vi "Compute Waveform.vi"(6 "signal type":T1, 8 "amplitude":dbl, 9 "phase increment":dbl, 10 "phase in":dbl, 11 "wfm size":i32) -> (2 "phase out":dbl, 3 "wfm array":dbl[](array[numeric]))   [LabVIEW 2023]
uses:
  Simulated Signal Type.ctl
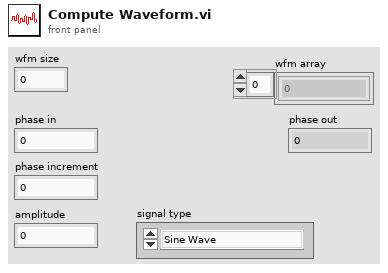
[diagram p1: front panel]
types:
  T1 = typedef "Simulated Signal Type.ctl" = enum16{"Sine Wave", "Square Wave with Noise"}
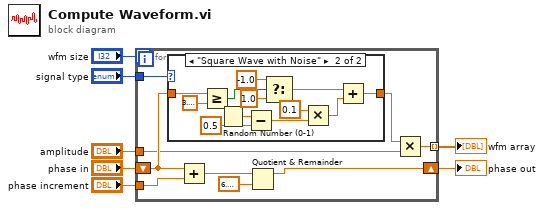
[diagram p0: block diagram]
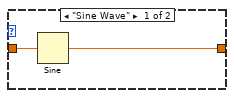
[diagram p2: hidden frame]
diagram:
  n1 = for {
    N: "wfm size" -> [_]
    tunnel: "signal type" -> [w8]
    tunnel: "phase increment" -> [w11]
    shift-right: [w14] -> w2
    shift-left: "phase in" -> [w16]
    tunnel: "amplitude" -> [w9]
    tunnel: [w10] -> w6 mode=indexing
    n2 = case shown="\"Square Wave with Noise\"" w8 {
      tunnel: w16 -> [w18 w30]
      tunnel: [w17 w22] -> w12
      frame "Sine Wave" {
        n3 = Sine(x=w18) -> (sin(x)=w17:dbl)
      }
      frame "Square Wave with Noise" {
        n4 = Greater Or Equal?(x=w30, y=3.141592653589793) -> (x >= y?=w27:bool)
        n5 = Random Number (0-1)() -> (number: 0 to 1=w24:dbl)
        n6 = Subtract(x=w24, y=0.5) -> (x-y=w21:dbl)
        n7 = Select(t=-1.0, s=w27, f=1.0 ("t")) -> (s? t:f=w28:dbl)
        n8 = Multiply(x=0.1, y=w21) -> (x*y=w20:dbl)
        n9 = Add(x=w28, y=w20) -> (x+y=w22:dbl)
      }
    }
    n10 = Add(x=w16, y=w11) -> (x+y=w15:dbl)
    n11 = Quotient & Remainder(x=w15, y=6.283185307179586) -> (x-y*floor(x/y)=w14:dbl)  [unwired: 1 out]
    n12 = Multiply(x=w12, y=w9) -> (x*y=w10:dbl)
  }
  "wfm array" <- w6
  "phase out" <- w2
